vi "Stop Processes.vi"(8 "error in (no error)":errorcluster, 11 "Execution UI In":refnum<class "Execution UI.lvclass">) -> (0 "error out":errorcluster, 3 "Execution UI Out":refnum<class "Execution UI.lvclass">)   [LabVIEW 2020, in "Execution UI.lvclass"]
uses:
  Execution UI.lvclass
  Execution UI.lvclass/Execution UI.ctl
  Helper Classes/Test Finder/Test Finder.lvclass
  Test Runner/Test Runner.lvclass
  Report Generator/Report Generator.lvclass
  Icon Decorator/Icon Decorator.lvclass
  Result Collector/Result Collector.lvclass
  Helper Classes/Test Result Tree/Test Result Tree.lvclass
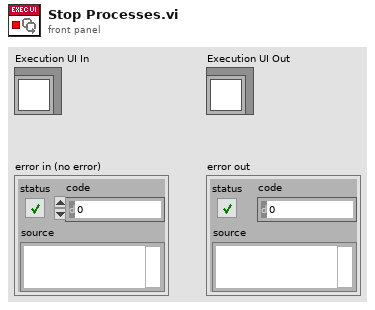
[diagram p1: front panel]
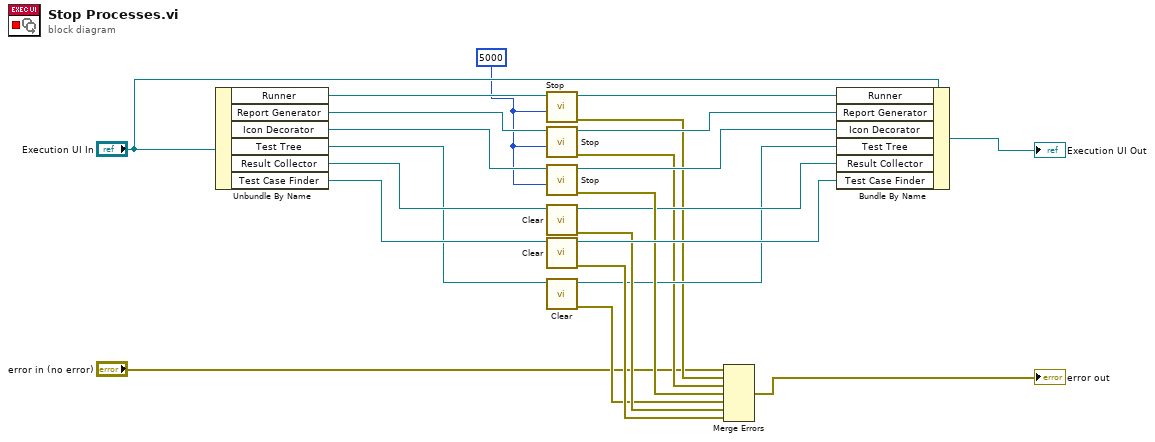
[diagram p0: block diagram]
diagram:
  w1 = 5000 ("timeout in ms (-1)")
  n1 = Unbundle By Name("Execution UI In") -> ("Runner"=w23:refnum<class "Test Runner.lvclass">, "Report Generator"=w5:refnum<class "Report Generator.lvclass">, "Icon Decorator"=w17:refnum<class "Icon Decorator.lvclass">, "Test Tree"=w13:refnum<class "Test Result Tree.lvclass">, "Result Collector"=w14:refnum<class "Result Collector.lvclass">, "Test Case Finder"=w21:refnum<class "Test Finder.lvclass">)
  n2 = call-dynamic "Stop.vi"("timeout in ms (-1)"=w1, "Test Runner In"=w23) -> ("error out"=w4:errorcluster, "Test Runner Out"=w9:refnum<class "Test Runner.lvclass">)  [unwired: 7 in, 1 out]
  n3 = call-dynamic "Stop.vi"("timeout in ms (-1)"=w1, "Process In"=w5) -> ("error out"=w6:errorcluster, "Process Out"=w8:refnum<class "Report Generator.lvclass">)  [unwired: 7 in, 1 out]
  n4 = call-dynamic "Stop.vi"("timeout in ms (-1)"=w1, "Process In"=w17) -> ("error out"=w19:errorcluster, "Process Out"=w18:refnum<class "Icon Decorator.lvclass">)  [unwired: 7 in, 1 out]
  n5 = call-dynamic "Clear.vi"("Report Generator In"=w14) -> ("error out"=w16:errorcluster, "Report Generator Out"=w15:refnum<class "Result Collector.lvclass">)  [unwired: 9 in]
  n6 = call "Clear.vi"("Test Finder in"=w21) -> ("error out"=w20:errorcluster, "Test Finder out"=w22:refnum<class "Test Finder.lvclass">)  [unwired: 9 in]
  n7 = call-dynamic "Clear.vi"("Test Tree In"=w13) -> ("error out"=w11:errorcluster, "Test Tree Out"=w12:refnum<class "Test Result Tree.lvclass">)  [unwired: 9 in]
  n8 = Merge Errors("error in (no error)", w4, w6, w19, w11, w16, w20) -> (→"error out":errorcluster)
  n9 = Bundle By Name(cluster="Execution UI In", "Runner"=w9, "Report Generator"=w8, "Icon Decorator"=w18, "Test Tree"=w12, "Result Collector"=w15, "Test Case Finder"=w22) -> (→"Execution UI Out":refnum<class "Execution UI.lvclass">)
